vi "Plot Current.vi"(7 "Current Mode":u8[](array[numeric]), 8 "XY Graph REF":refnum<vi>, 10 "plot setting":refnum<vi>) -> ()   [LabVIEW 2023]
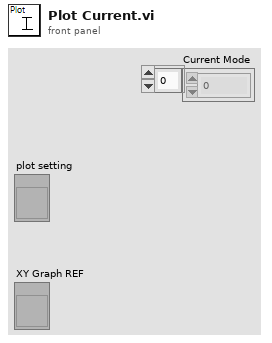
[diagram p1: front panel]
types:
  T1 = cluster{"V plot":bool, "I plot":bool, "Plot colour":u32, "Channel name\n":string}[]
  T2 = cluster{"V plot":bool, "I plot":bool, "Plot colour":u32, "Channel name\n":string}
  T3 = cluster{bool, "I plot":bool, "Plot colour":u32, "Channel name\n":string}
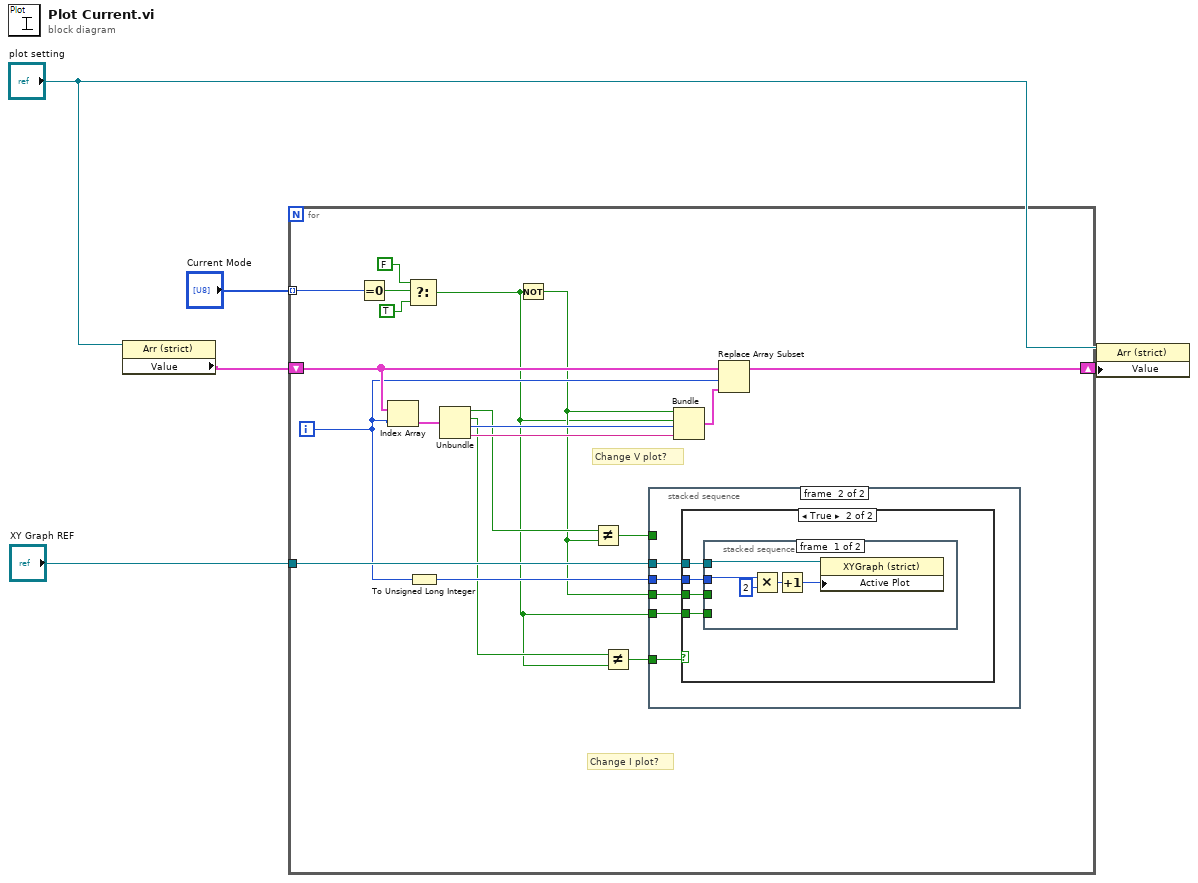
[diagram p0: block diagram]
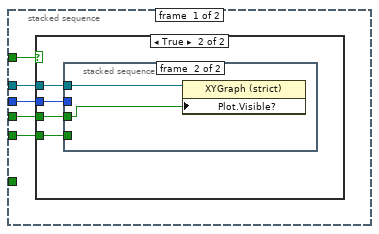
[diagram p2: hidden frame]
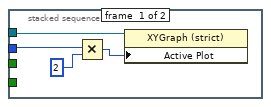
[diagram p4: hidden frame]
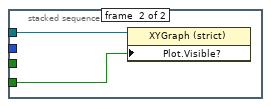
[diagram p6: hidden frame]
diagram:
  n1 = property class="Arr (strict)"(reference="plot setting") -> ("Value"=w3:T1)  [unwired: 1 in, 2 out]
  n2 = for {
    tunnel: "Current Mode" -> [w24] mode=indexing
    shift-right: [w15] -> w4
    shift-left: w3 -> [w20]
    tunnel: "XY Graph REF" -> [w14]
    i -> [w13]
    # "Change I plot?"
    # "Change V plot?"
    n3 = Equal To 0?(x=w24) -> (x = 0?=w23:bool)
    n4 = Index Array(array=w20, index=w13) -> (element=w19:T2)
    n5 = Select(t=FALSE ("I plot"), s=w23, f=TRUE ("I plot")) -> (s? t:f=w7:bool)
    n6 = To Unsigned Long Integer(number=w13) -> (unsigned 32bit integer=w12:u32)
    n7 = Unbundle(w19) -> ("V plot"=w11:bool, "I plot"=w8:bool, "Plot colour"=w18:u32, "Channel name"=w17:string)
    n8 = Not(x=w7) -> (.not. x?=w10:bool)
    n9 = Not Equal?(x=w11, y=w10) -> (x != y?=w9:bool)
    n10 = Not Equal?(x=w8, y=w7) -> (x != y?=w6:bool)
    n11 = stacked-sequence {
      tunnel: w14 -> [w29 w44]
      tunnel: w10 -> [w28 w43]
      tunnel: w12 -> [w27 w42]
      tunnel: w7 -> [w26 w41]
      tunnel: w9 -> [w25 _]
      tunnel: w6 -> [_ w40]
      frame #0 {
        n12 = case shown="True" w25 {
          tunnel: w29 -> [_ w33]
          tunnel: w28 -> [_ w32]
          tunnel: w27 -> [_ w31]
          tunnel: w26 -> [_ w30]
          frame False {
          }
          frame True {
            n13 = stacked-sequence {
              tunnel: w33 -> [w37 w39]
              tunnel: w31 -> [w34 _]
              tunnel: w32 -> [_ w38]
              tunnel: w30 -> [_ _]
              frame #0 {
                n14 = Multiply(x=w34, y=u32 2) -> (x*y=w35:u32)
                n15 = property class="XYGraph (strict)"(reference=w37, "Active Plot"=w35) -> ()  [unwired: 1 in, 2 out]
              }
              frame #1 {
                n16 = property class="XYGraph (strict)"(reference=w39, "Plot.Visible?"=w38) -> ()  [unwired: 1 in, 2 out]
              }
            }
          }
        }
      }
      frame #1 {
        n17 = case shown="True" w40 {
          tunnel: w44 -> [_ w48]
          tunnel: w43 -> [_ w47]
          tunnel: w42 -> [_ w46]
          tunnel: w41 -> [_ w45]
          frame False {
          }
          frame True {
            n18 = stacked-sequence {
              tunnel: w48 -> [w53 w55]
              tunnel: w46 -> [w49 _]
              tunnel: w47 -> [_ _]
              tunnel: w45 -> [_ w54]
              frame #0 {
                n19 = Multiply(x=w49, y=u32 2) -> (x*y=w51:u32)
                n20 = Increment(x=w51) -> (x+1=w50:u32)
                n21 = property class="XYGraph (strict)"(reference=w53, "Active Plot"=w50) -> ()  [unwired: 1 in, 2 out]
              }
              frame #1 {
                n22 = property class="XYGraph (strict)"(reference=w55, "Plot.Visible?"=w54) -> ()  [unwired: 1 in, 2 out]
              }
            }
          }
        }
      }
    }
    n23 = Bundle(w10, "I plot"=w7, "Plot colour"=w18, "Channel name"=w17) -> (w16:T3)  [unwired: 1 in]
    n24 = Replace Array Subset(array=w20, new element=w16, index=w13) -> (w15:T1)
  }
  n25 = property class="Arr (strict)"(reference="plot setting", "Value"=w4) -> ()  [unwired: 1 in, 2 out]
